vi "Send Command.vi"(8 "error in (no error)":errorcluster, 10 "Commands Enum":T1, 11 "Sensor General Class in":refnum<class "Sensor General Class.lvclass">) -> (0 "error out":errorcluster, 3 "Sensor General Class out":refnum<class "Sensor General Class.lvclass">)   [LabVIEW 2020, in "Sensor General Class.lvclass"]
uses:
  Sensor General Class.lvclass
  Commands Enum.ctl
  Sensor General Class.lvclass/Sensor General Class.ctl
  SubVI/MB Serial Master Query Write Single Register (poly).vi
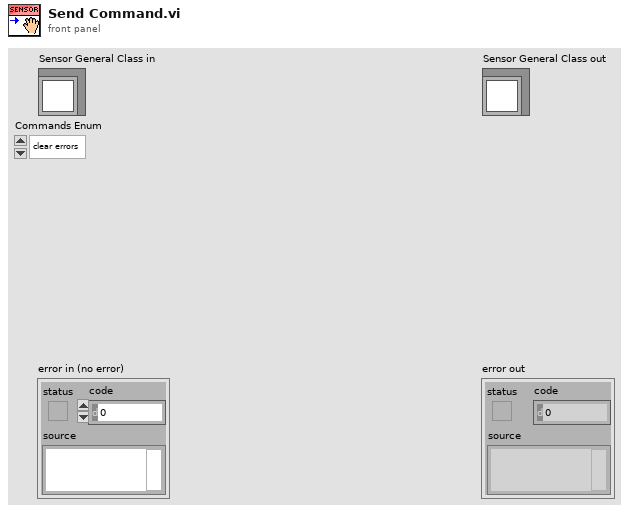
[diagram p1: front panel]
types:
  T1 = typedef "Sensor General Class.lvclass/Commands Enum.ctl" = enum16{"clear errors", "reset", "to default", "heat on", "service mode"}
  T2 = cluster{"Mode":enum16{"RTU", "ASCII"}, "Slave Address":u8}
  T3 = cluster{"index":i32, "name":string, "register":u16, "data":u16}[]
  T4 = cluster{"index":i32, "name":string, "register":u16, "data":u16}
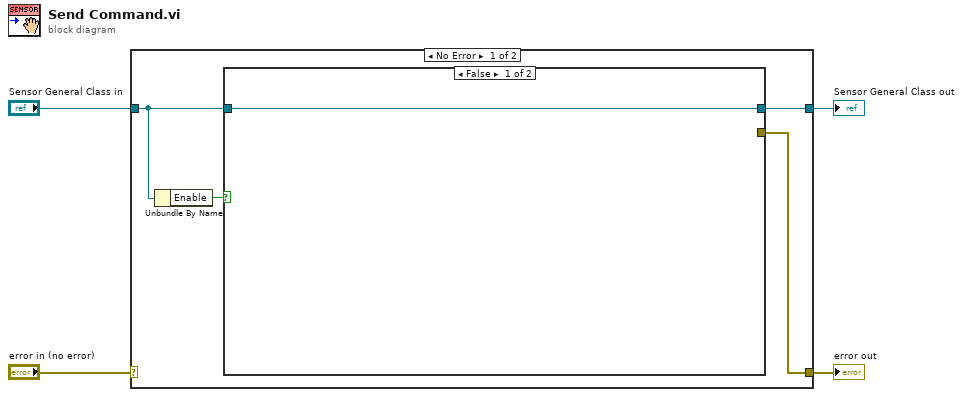
[diagram p0: block diagram]
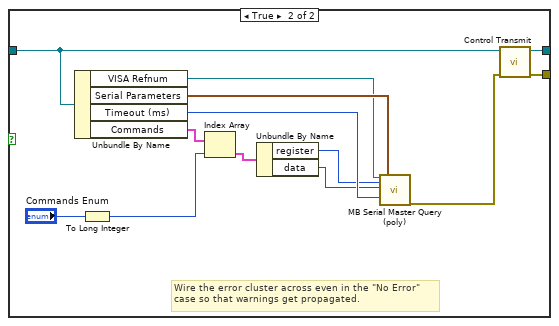
[diagram p2: hidden frame]
diagram:
  n1 = case shown="No Error" "error in (no error)" {
    selector: "error in (no error)" -> [_ w24]
    tunnel: [w7 w24] -> w3
    tunnel: [w8 w23] -> w1
    tunnel: "Sensor General Class in" -> [w6 w23]
    frame No Error {
      n2 = Unbundle By Name(w6) -> ("Enable"=w5:bool)
      n3 = case shown="False" w5 {
        tunnel: w6 -> [w9 w13]
        tunnel: [w9 w12] -> w8
        tunnel: [_ w10] -> w7
        frame False {
        }
        frame True {
          # "Wire the error cluster across even in the \"No Error\"\ncase so that warnings get propagated."
          n4 = Unbundle By Name(w13) -> ("VISA Refnum"=w21:refnum<visa-resource-name>, "Serial Parameters"=w22:T2, "Timeout (ms)"=w20:u32, "Commands"=w18:T3)
          n5 = To Long Integer(number="Commands Enum") -> (32bit integer=w17:i32)
          n6 = Index Array(array=w18, index=w17) -> (element=w16:T4)
          n7 = Unbundle By Name(w16) -> ("register"=w15:u16, "data"=w14:u16)
          n8 = call-poly <vilib>:"MB Serial Master Query (poly).vi"("VISA resource name"=w21, "Address"=w15, "Holding Register"=w14, "Timeout"=w20, "Serial Parameters"=w22) -> ("error out"=w11:errorcluster)  [unwired: 12 in, 2 out]
          n9 = call-dynamic "Control Transmit.vi"("error in (no error)"=w11, "Sensor General Class in"=w13) -> ("error out"=w10:errorcluster, "Sensor General Class out"=w12:refnum<class "Sensor General Class.lvclass">)  [unwired: 8 in]
        }
      }
    }
    frame Error {
    }
  }
  "error out" <- w3
  "Sensor General Class out" <- w1
